vi "Tx-RxFilt.vi"(0 "COMPORT":refnum<visa-resource-name>="COM4", 2 "REVC(T)":bool=TRUE, 3 "AntPort":i32=1 min=0 max=8 step=1, 5 "error in (no error)":errorcluster, 6 "RO(t)":bool, 7 "RX/TX":i32(ring)=1 items=["RX", "TX"], 8 "VERIFY(t)":bool, 9 "Filt(sel)":i32(ring) items=["OFF", "LOW", "MID", "HIGH"], 11 "Open Ser(t)":bool, 12 "milliseconds to wait":u32, 13 "Close Ser(t)":bool) -> (10 "filt(num)":i32=3, 14 "comport":refnum<visa-resource-name>="COM4", 19 "error out":errorcluster)   [LabVIEW 2018]
panel:
  out "after substring":string
  out "rcmd":string
  out "wcmd":string
  out "filt(name)":string="high"
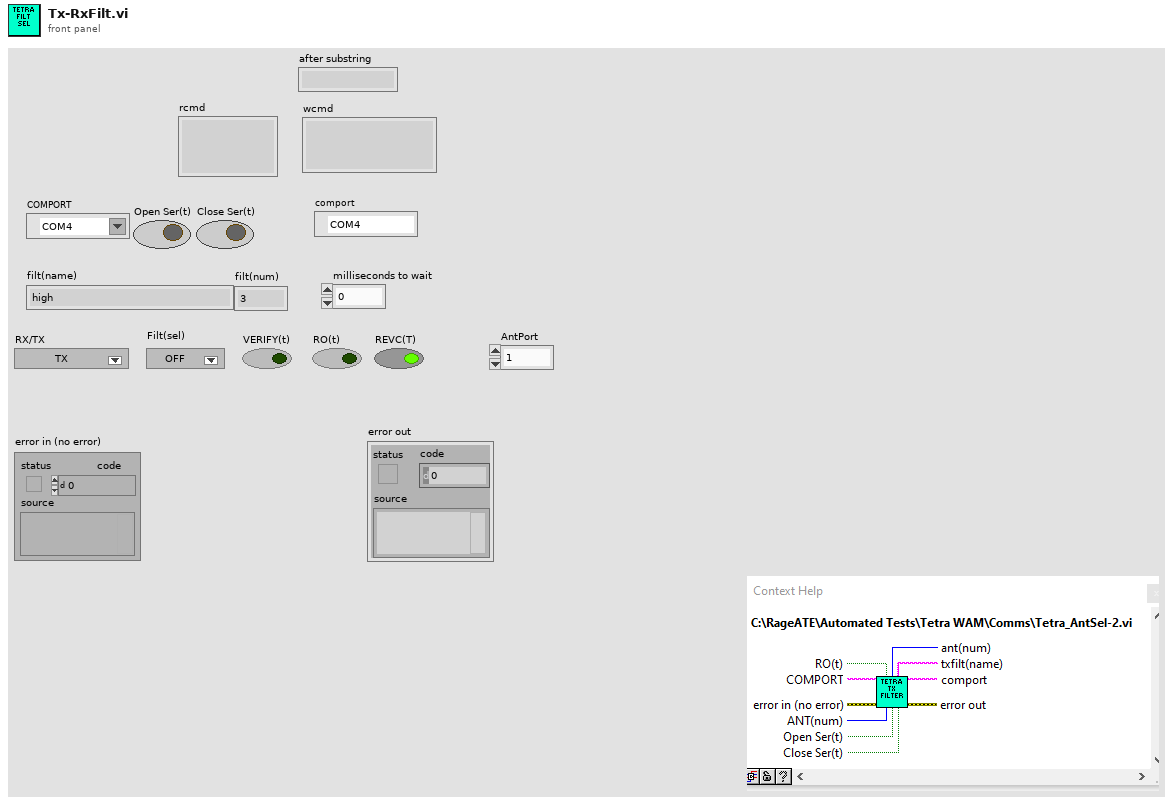
[diagram p1: front panel]
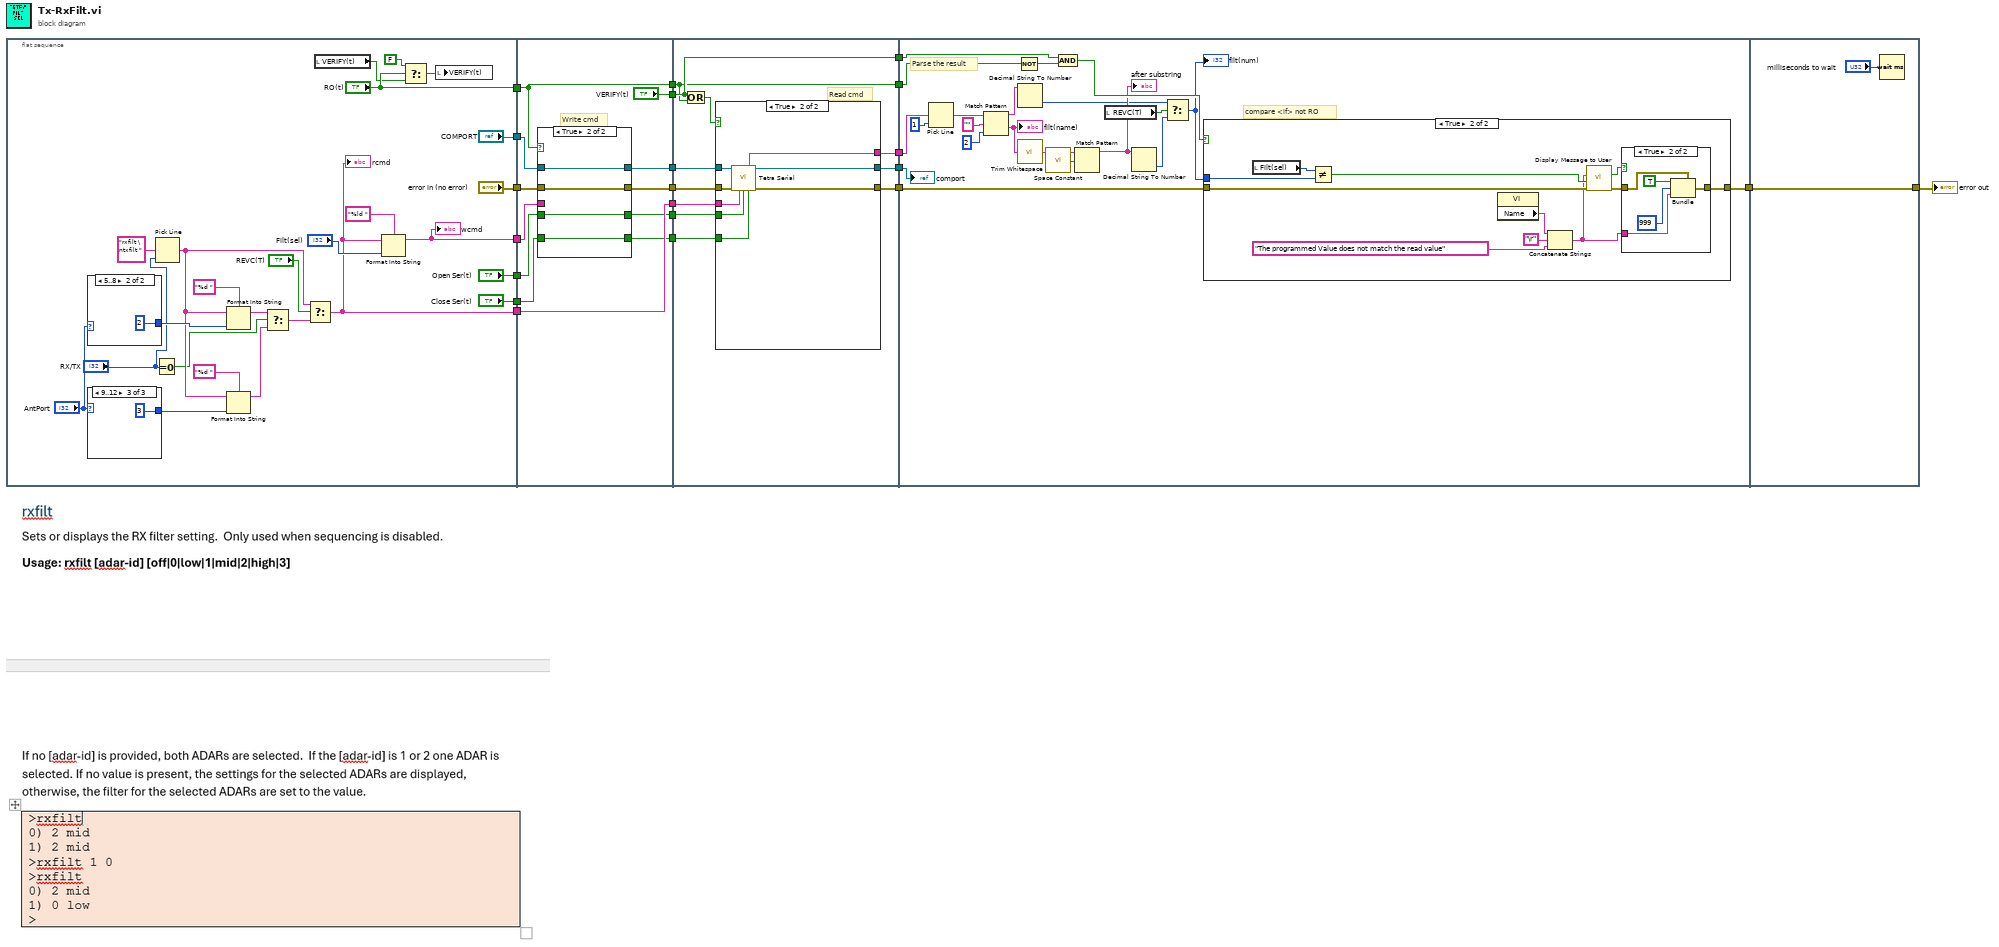
[diagram p0: block diagram]
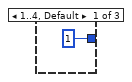
[diagram p2: hidden frame]
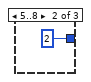
[diagram p3: hidden frame]
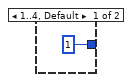
[diagram p4: hidden frame]
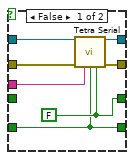
[diagram p5: hidden frame]
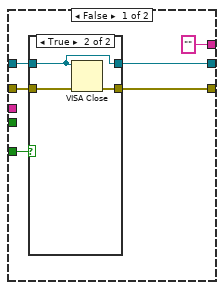
[diagram p6: hidden frame]
diagram:
  n1 = flat-sequence {
    tunnel: ["error in (no error)"] -> w21
    tunnel: ["COMPORT"] -> w20
    tunnel: [w39] -> w19
    tunnel: ["Open Ser(t)"] -> w18
    tunnel: [w38] -> w17
    tunnel: ["Close Ser(t)"] -> w16
    tunnel: ["RO(t)"] -> w9
    tunnel: w21 -> [w62]
    tunnel: w20 -> [w61]
    tunnel: w19 -> [w60]
    tunnel: w18 -> [w59]
    tunnel: w17 -> [w63]
    tunnel: w16 -> [w56]
    tunnel: [w63] -> w15
    tunnel: [w58] -> w14
    tunnel: [w57] -> w13
    tunnel: w9 -> [w53]
    tunnel: ["VERIFY(t)"] -> w8
    tunnel: [w55] -> w6
    tunnel: [w54] -> w5
    tunnel: [w53] -> w3
    tunnel: w15 -> [w75]
    tunnel: w14 -> [w84]
    tunnel: w13 -> [w85]
    tunnel: [w83] -> w12
    tunnel: [w82] -> w11
    tunnel: [w81] -> w10
    tunnel: w8 -> [w77]
    tunnel: [w77] -> w7
    tunnel: w6 -> [w80]
    tunnel: w5 -> [w79]
    tunnel: [w76] -> w4
    tunnel: w3 -> [w76]
    tunnel: w12 -> [w120]
    tunnel: w11 -> [w119]
    tunnel: w10 -> [w118]
    tunnel: w7 -> [w117]
    tunnel: w4 -> [w115]
    tunnel: [w113] -> w1
    tunnel: [w145] -> w2
    tunnel: w1 -> [w145]
    frame #0 {
      n2 = case shown="5..8" "AntPort" {
        tunnel: [1 ("input 1") 2 ("input 1")] -> w35
        frame 1..4, Default {
        }
        frame 5..8 {
        }
      }
      n3 = case shown="9..12" "AntPort" {
        tunnel: [1 ("input 1") 2 ("input 1") 3 ("input 1")] -> w33
        frame 1..4, Default {
        }
        frame 5..8 {
        }
        frame 9..12 {
        }
      }
      n4 = Equal To 0?(x="RX/TX") -> (x = 0?=w29:bool)
      n5 = Pick Line(multi-line string="rxfilt \ntxfilt ", line index="RX/TX") -> (output string=w32:string)  [unwired: 1 in]
      n6 = Format Into String(format string="%d ", initial string=w32, w35) -> (resulting string=w27:string)  [unwired: 1 in, 1 out]
      n7 = Format Into String(format string="%d ", initial string=w32, w33) -> (resulting string=w26:string)  [unwired: 1 in, 1 out]
      n8 = Select(t=w27, s=w29, f=w26) -> (s? t:f=w28:string)
      n9 = Select(t=w32, s="REVC(T)", f=w28) -> (s? t:f=w38:string)
      "rcmd" <- w38
      n10 = local read "VERIFY(t)"() -> (w22:bool)
      n11 = Format Into String(format string="%ld ", initial string=w38, "Filt(sel)") -> (resulting string=w39:string)  [unwired: 1 in, 1 out]
      "wcmd" <- w39
      n12 = Select(t=FALSE, s="RO(t)", f=w22) -> (s? t:f=w23:bool)
      n13 = local write "VERIFY(t)"(w23) -> ()
    }
    frame #1 {
      # "Write cmd"
      n14 = case shown="True" w53 {
        tunnel: w62 -> [w70 w74]
        tunnel: w61 -> [w69 w73]
        tunnel: w60 -> [w68 _]
        tunnel: w59 -> [_ w71]
        tunnel: [w67 w74] -> w58
        tunnel: [w66 w73] -> w57
        tunnel: w56 -> [w64 w72]
        tunnel: [w64 w72] -> w54
        tunnel: [w65 w71] -> w55
        frame False {
          w65 = FALSE
          n15 = call "Tetra Serial.vi"("COMPORT"=w69, "error in (no error)"=w70, "Command"=w68, "Open Ser(t)"=w64, "Close Ser(t)"=w65) -> ("comport"=w66:refnum<visa-resource-name>, "error out"=w67:errorcluster)  [unwired: 6 in, 3 out]
        }
        frame True {
        }
      }
    }
    frame #2 {
      # "Read cmd"
      n16 = Or(x=w77, y=w76) -> (x .or. y?=w78:bool)
      n17 = case shown="True" w78 {
        tunnel: w85 -> [w90 w104]
        tunnel: w84 -> [w88 w103]
        tunnel: w75 -> [_ w102]
        tunnel: ["" ("output") w101] -> w83
        tunnel: [w86 w100] -> w82
        tunnel: [w89 w99] -> w81
        tunnel: w80 -> [_ w98]
        tunnel: w79 -> [w87 w97]
        frame False {
          n18 = case shown="True" w87 {
            tunnel: w90 -> [w92 w94]
            tunnel: [w93 w96] -> w89
            tunnel: w88 -> [w93 w95]
            tunnel: [w92 w94] -> w86
            frame False {
            }
            frame True {
              n19 = VISA Close(VISA resource name=w94, error in (no error)=w95) -> (error out=w96:errorcluster)
            }
          }
        }
        frame True {
          n20 = call "Tetra Serial.vi"("COMPORT"=w104, "error in (no error)"=w103, "Command"=w102, "Open Ser(t)"=w98, "Close Ser(t)"=w97) -> ("output"=w101:string, "comport"=w100:refnum<visa-resource-name>, "error out"=w99:errorcluster)  [unwired: 6 in, 2 out]
        }
      }
    }
    frame #3 {
      # "Parse the result"
      # "compare <if> not RO"
      n21 = Pick Line(multi-line string=w120, line index=1) -> (output string=w124:string)  [unwired: 1 in]
      n22 = Match Pattern(string=w124, regular expression="", offset (0)=2) -> (before substring=w125:string, after substring=w112:string)  [unwired: 2 out]
      "filt(name)" <- w112
      n23 = Not(x=w115) -> (.not. x?=w116:bool)
      n24 = Decimal String To Number(string=w125) -> (number=w107:i32)  [unwired: 2 in, 1 out]
      n25 = call <vilib>:"Trim Whitespace.vi"("string"=w112) -> ("trimmed string"=w111:string)  [unwired: 1 in]
      n26 = call <vilib>:"Space Constant.vi"() -> ("String"=w110:string)
      n27 = And(x=w117, y=w116) -> (x .and. y?=w114:bool)
      n28 = Match Pattern(string=w111, regular expression=w110) -> (before substring=w109:string)  [unwired: 1 in, 3 out]
      "after substring" <- w109
      n29 = local read "REVC(T)"() -> (w108:bool)
      n30 = Decimal String To Number(string=w109) -> (number=w105:i32)  [unwired: 2 in, 1 out]
      n31 = Select(t=w107, s=w108, f=w105) -> (s? t:f=w106:i32)
      "filt(num)" <- w106
      n32 = case shown="True" w114 {
        tunnel: w106 -> [_ w137]
        tunnel: w118 -> [w126 w136]
        tunnel: [w126 w134] -> w113
        frame False {
        }
        frame True {
          n33 = local read "Filt(sel)"() -> (w127:i32)
          n34 = Not Equal?(x=w127, y=w137) -> (x != y?=w132:bool)
          n35 = property class="VI"() -> ("Name"=w133:string)  [unwired: 2 in, 2 out]
          n36 = Concatenate Strings(w133, "\r", "The programmed Value does not match the read value" ("Message")) -> (w130:string)
          n37 = call "Display Message to User"("error in (no error)"=w136, "Enable"=w132, "Message"=w130) -> ("error out"=w135:errorcluster, "OK"=w131:bool)  [unwired: 7 in]
          n38 = case shown="True" w131 {
            tunnel: w135 -> [w138 w142]
            tunnel: [w138 w143] -> w134
            tunnel: w130 -> [_ w141]
            frame False {
            }
            frame True {
              n39 = Bundle(cluster=w142, "status"=TRUE, "code"=999, "source"=w141) -> (w143:errorcluster)
            }
          }
        }
      }
      "comport" <- w119
    }
    frame #4 {
      n40 = Wait (ms)(milliseconds to wait="milliseconds to wait") -> ()  [unwired: 1 out]
    }
  }
  "error out" <- w2
